vi "Constants.vi"() -> ()   [LabVIEW 2020, in "NI_VS Data Logging API.lvlib"]
doc: "Contains constants used by the NI_VS Data Logging API library."
uses:
  <vilib>/NI VeriStand/Execution/DataLogging/NI_VS Data Logging API.lvlib
panel:
  in  "Invalid Property Error":i32=-307863
  in  "Invalid Property Type (%s %s)":string="The specified value is not a valid data type for a TDMS property.\n\nProperty name: %s\nSpecified data type: %s\n\nYou must specify a value from one of the following data types: I8, I16, I32, I64, U8, U16, U32, U64, Single, Double, String, Timestamp, Boolean."
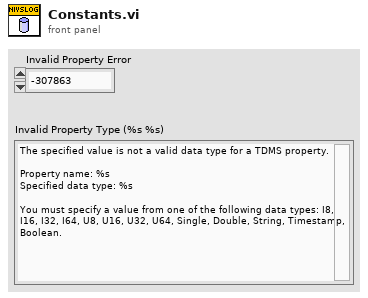
[diagram p1: front panel]
diagram:
